vi "test_LoadCommandlineArgs.vi"() -> (3 "Pass?":bool)   [LabVIEW 2020, in "Tests.SolutionBuilder.lvlib"]
uses:
  Tests.SolutionBuilder.lvlib
  SolutionBuilder/Community/Options.ctl
  SolutionBuilder/ProjectItem/ProjectItem.lvclass
  SolutionBuilder/SolutionBuilder.lvclass
panel:
  out "test results":u32 format="%014b"
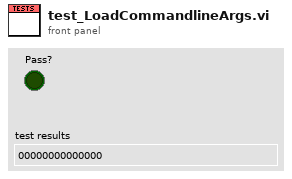
[diagram p1: front panel]
types:
  T1 = typedef "SolutionBuilder.lvlib/SolutionBuilder.lvclass/Options.ctl" = cluster{"Path":path, "Preview?":bool, "Quiet?":bool, "Log file":path, "Success file":path}
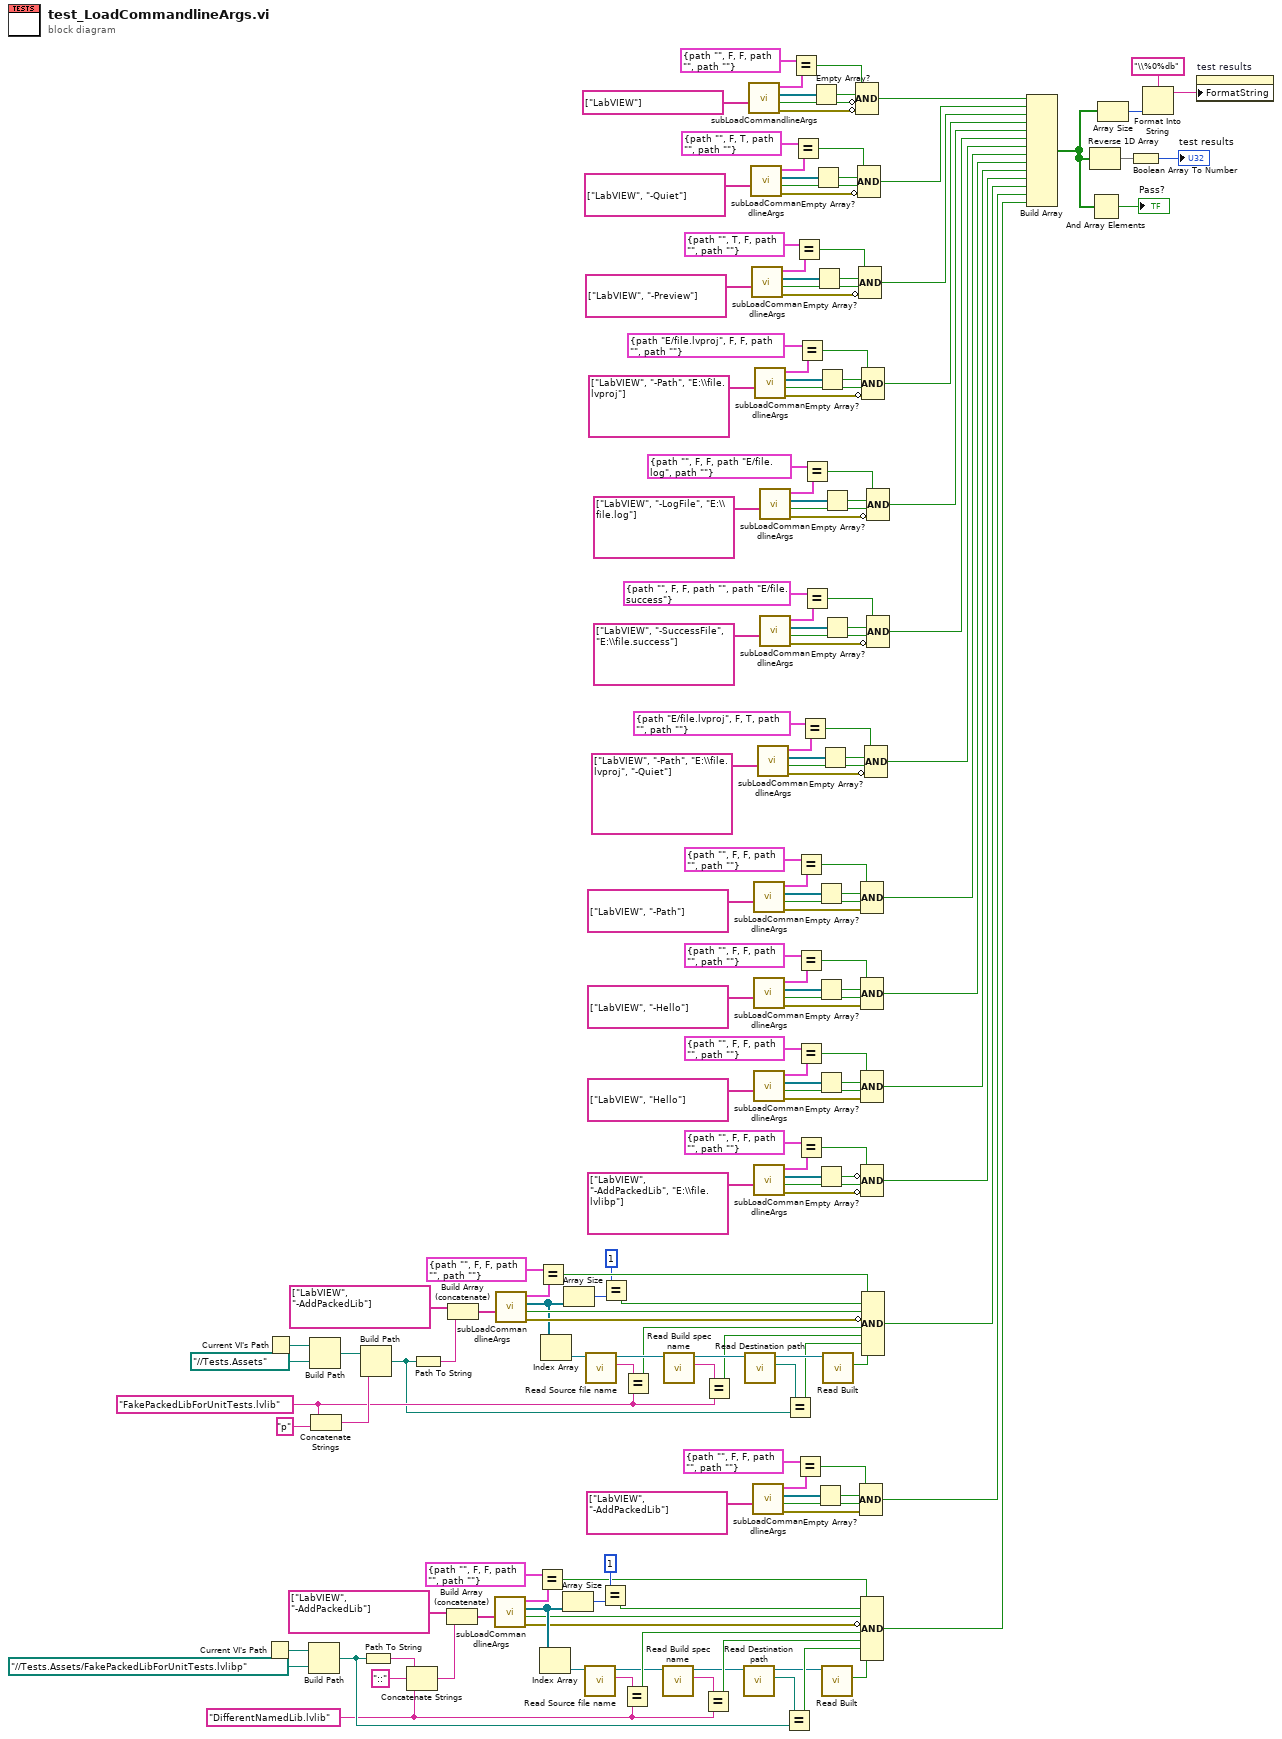
[diagram p0: block diagram]
diagram:
  w31 = "DifferentNamedLib.lvlib" ("string")
  w65 = "FakePackedLibForUnitTests.lvlib"
  n1 = Current VI's Path() -> (path=w46:path)
  n2 = Current VI's Path() -> (path=w79:path)
  n3 = Build Path(base path=w46, name or relative path=path "../../Tests.Assets/FakePackedLibForUnitTests.lvlibp" ("Path")) -> (appended path=w35:path)
  n4 = Build Path(base path=w79, name or relative path=path "../../Tests.Assets" ("Path")) -> (appended path=w75:path)
  n5 = Concatenate Strings(w65, "p" ("string")) -> (w72:string)
  n6 = Build Path(base path=w75, name or relative path=w72) -> (appended path=w64:path)
  n7 = Path To String(path=w35) -> (string=w33:string)
  n8 = Concatenate Strings(w33, "::" ("string"), w31) -> (w32:string)
  n9 = Path To String(path=w64) -> (string=w77:string)
  n10 = Build Array (concatenate)(string[] ["LabVIEW", "-AddPackedLib"] ("App.Args"), w32) -> (w47:string[])
  n11 = Build Array (concatenate)(string[] ["LabVIEW", "-AddPackedLib"] ("App.Args"), w77) -> (w78:string[])
  n12 = call "subLoadCommandlineArgs.vi"("App.Args"=w47) -> ("error out"=w41:errorcluster, "From command line?"=w37:bool, "Pre-built libraries"=w48:refnum<class "ProjectItem.lvclass">[], "Options"=w39:T1)  [unwired: 7 in]
  n13 = call "subLoadCommandlineArgs.vi"("App.Args"=w78) -> ("error out"=w101:errorcluster, "From command line?"=w105:bool, "Pre-built libraries"=w76:refnum<class "ProjectItem.lvclass">[], "Options"=w103:T1)  [unwired: 7 in]
  n14 = Equal?(x=T1 {"Path"=path "", "Preview?"=FALSE, "Quiet?"=FALSE, "Log file"=path "", "Success file"=path ""} ("Options"), y=w39) -> (x = y?=w38:bool)
  n15 = Equal?(x=T1 {"Path"=path "", "Preview?"=FALSE, "Quiet?"=FALSE, "Log file"=path "", "Success file"=path ""} ("Options"), y=w103) -> (x = y?=w104:bool)
  n16 = Index Array(array=w48) -> (element=w49:refnum<class "ProjectItem.lvclass">)  [unwired: 1 in]
  n17 = Index Array(array=w76) -> (element=w74:refnum<class "ProjectItem.lvclass">)  [unwired: 1 in]
  n18 = Array Size(array=w48) -> (size(s)=w42:i32)
  n19 = Array Size(array=w76) -> (size(s)=w100:i32)
  n20 = call-dynamic "Read Source file name.vi"("ProjectItem in"=w49) -> ("Source file name"=w54:string, "ProjectItem out"=w50:refnum<class "ProjectItem.lvclass">)  [unwired: 9 in]
  n21 = call-dynamic "Read Source file name.vi"("ProjectItem in"=w74) -> ("Source file name"=w67:string, "ProjectItem out"=w71:refnum<class "ProjectItem.lvclass">)  [unwired: 9 in]
  n22 = Equal?(x=1, y=w42) -> (x = y?=w44:bool)
  n23 = Equal?(x=1, y=w100) -> (x = y?=w98:bool)
  n24 = Equal?(x=w54, y=w31) -> (x = y?=w57:bool)
  n25 = Equal?(x=w67, y=w65) -> (x = y?=w62:bool)
  n26 = call-dynamic "Read Build spec name.vi"("ProjectItem in"=w50) -> ("Build spec name"=w55:string, "ProjectItem out"=w51:refnum<class "ProjectItem.lvclass">)  [unwired: 9 in]
  n27 = call-dynamic "Read Build spec name.vi"("ProjectItem in"=w71) -> ("Build spec name"=w66:string, "ProjectItem out"=w70:refnum<class "ProjectItem.lvclass">)  [unwired: 9 in]
  n28 = Equal?(x=w55, y=w31) -> (x = y?=w58:bool)
  n29 = Equal?(x=w66, y=w65) -> (x = y?=w61:bool)
  n30 = call-dynamic "Read Destination path.vi"("ProjectItem in"=w51) -> ("Destination path"=w56:path, "ProjectItem out"=w52:refnum<class "ProjectItem.lvclass">)  [unwired: 9 in]
  n31 = call-dynamic "Read Destination path.vi"("ProjectItem in"=w70) -> ("Destination path"=w63:path, "ProjectItem out"=w69:refnum<class "ProjectItem.lvclass">)  [unwired: 9 in]
  n32 = call "subLoadCommandlineArgs.vi"("App.Args"=string[] ["LabVIEW"]) -> ("error out"=w144:errorcluster, "From command line?"=w170:bool, "Pre-built libraries"=w173:refnum<class "ProjectItem.lvclass">[], "Options"=w175:T1)  [unwired: 7 in]
  n33 = call "subLoadCommandlineArgs.vi"("App.Args"=string[] ["LabVIEW", "-Quiet"]) -> ("error out"=w145:errorcluster, "From command line?"=w166:bool, "Pre-built libraries"=w163:refnum<class "ProjectItem.lvclass">[], "Options"=w162:T1)  [unwired: 7 in]
  n34 = call "subLoadCommandlineArgs.vi"("App.Args"=string[] ["LabVIEW", "-Preview"]) -> ("error out"=w146:errorcluster, "From command line?"=w154:bool, "Pre-built libraries"=w157:refnum<class "ProjectItem.lvclass">[], "Options"=w158:T1)  [unwired: 7 in]
  n35 = call "subLoadCommandlineArgs.vi"("App.Args"=string[] ["LabVIEW", "-AddPackedLib"]) -> ("error out"=w91:errorcluster, "From command line?"=w97:bool, "Pre-built libraries"=w94:refnum<class "ProjectItem.lvclass">[], "Options"=w93:T1)  [unwired: 7 in]
  n36 = call "subLoadCommandlineArgs.vi"("App.Args"=string[] ["LabVIEW", "-Path"]) -> ("error out"=w137:errorcluster, "From command line?"=w131:bool, "Pre-built libraries"=w134:refnum<class "ProjectItem.lvclass">[], "Options"=w135:T1)  [unwired: 7 in]
  n37 = call "subLoadCommandlineArgs.vi"("App.Args"=string[] ["LabVIEW", "-Hello"]) -> ("error out"=w115:errorcluster, "From command line?"=w121:bool, "Pre-built libraries"=w118:refnum<class "ProjectItem.lvclass">[], "Options"=w117:T1)  [unwired: 7 in]
  n38 = call "subLoadCommandlineArgs.vi"("App.Args"=string[] ["LabVIEW", "Hello"]) -> ("error out"=w114:errorcluster, "From command line?"=w108:bool, "Pre-built libraries"=w111:refnum<class "ProjectItem.lvclass">[], "Options"=w112:T1)  [unwired: 7 in]
  n39 = call "subLoadCommandlineArgs.vi"("App.Args"=string[] ["LabVIEW", "-AddPackedLib", "E:\\file.lvlibp"]) -> ("error out"=w82:errorcluster, "From command line?"=w88:bool, "Pre-built libraries"=w85:refnum<class "ProjectItem.lvclass">[], "Options"=w84:T1)  [unwired: 7 in]
  n40 = call "subLoadCommandlineArgs.vi"("App.Args"=string[] ["LabVIEW", "-Path", "E:\\file.lvproj"]) -> ("error out"=w143:errorcluster, "From command line?"=w152:bool, "Pre-built libraries"=w149:refnum<class "ProjectItem.lvclass">[], "Options"=w148:T1)  [unwired: 7 in]
  n41 = call "subLoadCommandlineArgs.vi"("App.Args"=string[] ["LabVIEW", "-Path", "E:\\file.lvproj", "-Quiet"]) -> ("error out"=w130:errorcluster, "From command line?"=w124:bool, "Pre-built libraries"=w127:refnum<class "ProjectItem.lvclass">[], "Options"=w128:T1)  [unwired: 7 in]
  n42 = call "subLoadCommandlineArgs.vi"("App.Args"=string[] ["LabVIEW", "-LogFile", "E:\\file.log"]) -> ("error out"=w17:errorcluster, "From command line?"=w11:bool, "Pre-built libraries"=w14:refnum<class "ProjectItem.lvclass">[], "Options"=w15:T1)  [unwired: 7 in]
  n43 = call "subLoadCommandlineArgs.vi"("App.Args"=string[] ["LabVIEW", "-SuccessFile", "E:\\file.success"]) -> ("error out"=w4:errorcluster, "From command line?"=w10:bool, "Pre-built libraries"=w7:refnum<class "ProjectItem.lvclass">[], "Options"=w6:T1)  [unwired: 7 in]
  n44 = Equal?(x=w56, y=w35) -> (x = y?=w59:bool)
  n45 = Equal?(x=w63, y=w64) -> (x = y?=w60:bool)
  n46 = Equal?(x=T1 {"Path"=path "", "Preview?"=FALSE, "Quiet?"=FALSE, "Log file"=path "", "Success file"=path ""} ("Options"), y=w175) -> (x = y?=w171:bool)
  n47 = Equal?(x=T1 {"Path"=path "", "Preview?"=FALSE, "Quiet?"=TRUE, "Log file"=path "", "Success file"=path ""} ("Options"), y=w162) -> (x = y?=w165:bool)
  n48 = Equal?(x=T1 {"Path"=path "", "Preview?"=TRUE, "Quiet?"=FALSE, "Log file"=path "", "Success file"=path ""} ("Options"), y=w158) -> (x = y?=w155:bool)
  n49 = Equal?(x=T1 {"Path"=path "", "Preview?"=FALSE, "Quiet?"=FALSE, "Log file"=path "", "Success file"=path ""} ("Options"), y=w93) -> (x = y?=w96:bool)
  n50 = Equal?(x=T1 {"Path"=path "", "Preview?"=FALSE, "Quiet?"=FALSE, "Log file"=path "", "Success file"=path ""} ("Options"), y=w135) -> (x = y?=w132:bool)
  n51 = Equal?(x=T1 {"Path"=path "", "Preview?"=FALSE, "Quiet?"=FALSE, "Log file"=path "", "Success file"=path ""} ("Options"), y=w117) -> (x = y?=w120:bool)
  n52 = Equal?(x=T1 {"Path"=path "", "Preview?"=FALSE, "Quiet?"=FALSE, "Log file"=path "", "Success file"=path ""} ("Options"), y=w112) -> (x = y?=w109:bool)
  n53 = Equal?(x=T1 {"Path"=path "", "Preview?"=FALSE, "Quiet?"=FALSE, "Log file"=path "", "Success file"=path ""} ("Options"), y=w84) -> (x = y?=w87:bool)
  n54 = Equal?(x=T1 {"Path"=path "E:/file.lvproj", "Preview?"=FALSE, "Quiet?"=FALSE, "Log file"=path "", "Success file"=path ""} ("Options"), y=w148) -> (x = y?=w151:bool)
  n55 = Equal?(x=T1 {"Path"=path "E:/file.lvproj", "Preview?"=FALSE, "Quiet?"=TRUE, "Log file"=path "", "Success file"=path ""} ("Options"), y=w128) -> (x = y?=w125:bool)
  n56 = Equal?(x=T1 {"Path"=path "", "Preview?"=FALSE, "Quiet?"=FALSE, "Log file"=path "E:/file.log", "Success file"=path ""} ("Options"), y=w15) -> (x = y?=w12:bool)
  n57 = Equal?(x=T1 {"Path"=path "", "Preview?"=FALSE, "Quiet?"=FALSE, "Log file"=path "", "Success file"=path "E:/file.success"} ("Options"), y=w6) -> (x = y?=w9:bool)
  n58 = Empty Array?(array=w173) -> (empty?=w172:bool)
  n59 = Empty Array?(array=w163) -> (empty?=w164:bool)
  n60 = Empty Array?(array=w157) -> (empty?=w156:bool)
  n61 = Empty Array?(array=w94) -> (empty?=w95:bool)
  n62 = Empty Array?(array=w134) -> (empty?=w133:bool)
  n63 = Empty Array?(array=w118) -> (empty?=w119:bool)
  n64 = Empty Array?(array=w111) -> (empty?=w110:bool)
  n65 = Empty Array?(array=w85) -> (empty?=w86:bool)
  n66 = Empty Array?(array=w149) -> (empty?=w150:bool)
  n67 = Empty Array?(array=w127) -> (empty?=w126:bool)
  n68 = Empty Array?(array=w14) -> (empty?=w13:bool)
  n69 = Empty Array?(array=w7) -> (empty?=w8:bool)
  n70 = call-dynamic "Read Built.vi"("ProjectItem in"=w52) -> ("Built"=w53:bool)  [unwired: 9 in, 1 out]
  n71 = call-dynamic "Read Built.vi"("ProjectItem in"=w69) -> ("Built"=w68:bool)  [unwired: 9 in, 1 out]
  n72 = Compound Arithmetic op=AND(w171, w172, invert w170, invert w144) -> (w169:bool)
  n73 = Compound Arithmetic op=AND(w165, w164, w166, invert w145) -> (w160:bool)
  n74 = Compound Arithmetic op=AND(w155, w156, w154, invert w146) -> (w153:bool)
  n75 = Compound Arithmetic op=AND(w96, w95, w97, w91) -> (w89:bool)
  n76 = Compound Arithmetic op=AND(w132, w133, w131, w137) -> (w122:bool)
  n77 = Compound Arithmetic op=AND(w120, w119, w121, w115) -> (w107:bool)
  n78 = Compound Arithmetic op=AND(w109, w110, w108, w114) -> (w106:bool)
  n79 = Compound Arithmetic op=AND(w87, invert w86, w88, invert w82) -> (w81:bool)
  n80 = Compound Arithmetic op=AND(w38, w44, w37, invert w41, w57, w58, w59, w53) -> (w36:bool)
  n81 = Compound Arithmetic op=AND(w151, w150, w152, invert w143) -> (w142:bool)
  n82 = Compound Arithmetic op=AND(w104, w98, w105, invert w101, w62, w61, w60, w68) -> (w90:bool)
  n83 = Compound Arithmetic op=AND(w125, w126, w124, invert w130) -> (w123:bool)
  n84 = Compound Arithmetic op=AND(w12, w13, w11, invert w17) -> (w2:bool)
  n85 = Compound Arithmetic op=AND(w9, w8, w10, invert w4) -> (w1:bool)
  n86 = Build Array(w169, w160, w153, w142, w2, w1, w123, w122, w107, w106, w81, w90, w89, w36) -> (w141:bool[])
  n87 = Reverse 1D Array(array=w141) -> (reversed array=w30:bool[])
  n88 = And Array Elements(Boolean array=w141) -> (logical AND=→"Pass?":bool)
  n89 = Array Size(array=w141) -> (size(s)=w139:i32)
  n90 = Boolean Array To Number(Boolean array=w30) -> (number=→"test results":u32)
  n91 = Format Into String(format string="\\%0%db", w139) -> (resulting string=w138:string)  [unwired: 2 in, 1 out]
  n92 = property on="test results" class="DigNum (strict)"("FormatString"=w138) -> ()  [unwired: 2 in, 2 out]
